vi "Joystick_Operation.vi"(0 "System no.":i32=1 min=1 max=4 step=1, 1 "Joystick ID":u32, 2 "X axis":string="B", 3 "Y axis":string="E", 4 "No.of digits for MOV command":i16=2, 5 "error in":errorcluster, 6 "Resolution factor X":i32=150, 7 "Resolution factor Y":i32=150, 8 "Dead band X":i32=2, 9 "Dead band Y":i32=2, 10 "Use #24 for Stop?":bool=TRUE, 11 "Read from controller?":bool=TRUE caption="Read travel range\nfrom controller?", 12 "Maximum velocity values":T2={"Velocity1 X"=1.0, "Velocity2 X"=20.0, "Velocity1 Y"=0.5, "Velocity2 Y"=15.0} {"Velocity2 Y" format="%.6f"; "Velocity1 Y" format="%.6f"; "Velocity2 X" format="%.6f"; "Velocity1 X" format="%.6f"}, 13 "Travel range":T1={"Xmax"=10.0, "Xmin"=0.0, "Ymax"=5.0, "Ymin"=0.0} {"Ymin" format="%.6f"; "Ymax" format="%.6f"; "Xmin" format="%.6f"; "Xmax" format="%.6f"}, 14 "System no. 2":i32=1 min=1 max=4 step=1) -> (19 "error out":errorcluster)   [LabVIEW 2015]
doc: "This VI can be used to control 2 closed-loop axes (which can belong to one or two connected systems) with a standard 2-button, 2-axis joystick connected to the game port of the host computer. The absolute value of the joystick position is converted into a velocity values for the two stages connected to the system being commanded. Two velocity levels for each axis can be specified, e.g. one for fast, rough positioning and one for slow, fine positioning. Joystick button 2 switches between these levels. The sign of the joystick position determines whether the move command issued contains the positive or negative travel limit (read automatically if Read travel range from controller? is TRUE) of the corresponding axis. When the joystick is \"in the middle position\", the velocity of the corresponding axis is set to zero. \nDead band * is the maximum size of the scaled joystick position value that does not result in any motion. \nResolution factor * determines the joystick resolution. \nNo. of digits is the number of digits after the decimal point in the position values that will be sent by the MOV command. \nIf joystick button 1 is pressed, a stop command (STP or #24, depending on Use 24 for stop, is sent to the controller. The diagram shows how to combine the driver and support VIs for these tasks. \n\nIf only one motion axis is to be controlled, Y Axis must be identical to X Axis, System no. 2 must be identical to System no. 1, and Y axis of joystick is to be used for control of the motion axis.\n\nImportant: Install joystick driver and calibrate joystick in the Windows control panel before running this VI.\n\nValid for C-702, C-843, C-843.PM, C-844, C-848, C-865, C-866, C-867, C-880, E-710, E-712, E-725, E-753, E-755, E-761, E-861\n\nC-702: Use #24 for stop = TRUE, Read from controller = TRUE\n Run \"C702_Configuration_Setup.vi\" prior to running this VI.\n\nC-843: Use #24 for stop = TRUE, Read from controller = TRUE; \n Run \"C843_Configuration_Setup.vi\" prior to running this VI.\n\nC-843.PM: Use #24 for stop = TRUE, Read from controller = TRUE; \n Run \"C843_PM_Configuration_Setup.vi\" prior to running this VI.\n\nC-844: Use #24 for stop = TRUE, Read from controller = TRUE\n Run \"C844_Configuration_Setup.vi\" prior to running this VI.\n\nC-848: Use #24 for stop = TRUE, Read from controller = TRUE\n Run \"C848_Configuration_Setup.vi\" prior to running this VI.\n\nC-865: Use #24 for stop = TRUE, Read from controller = TRUE; \n Run \"C865_Configuration_Setup.vi\" prior to running this VI. \n\nC-866: Use #24 for stop = TRUE, Read from controller = TRUE; \n Run \"C866_Configuration_Setup.vi\" prior to running this VI. \n\nC-867: Use #24 for stop = TRUE, Read from controller = TRUE; \n Run \"C867_Configuration_Setup.vi\" prior to running this VI. \n\nC-880: Use #24 for stop = TRUE, Read from controller = TRUE\n Run \"C880_Configuration_Setup.vi\" prior to running this VI.\n\nE-710: Use #24 for stop = FALSE, Read from controller = TRUE. Default position unit is µm, default velocity unit is µm/ms. Joystick button 1 is not supported (controller does not support #24 or STP). Run \"E710_Configuration_Setup.vi\" prior to running this VI.\n\nE-712: Use #24 for stop = TRUE, Read from controller = TRUE. Default position unit is µm, default velocity unit is µm/s. Run \"E712_Configuration_Setup.vi\" prior to running this VI. \n\nE-725: Use #24 for stop = TRUE, Read from controller = TRUE. Default position unit is µm, default velocity unit is µm/s. Run \"E725_Configuration_Setup.vi\" prior to running this VI. \n\nE-753: Use #24 for stop = TRUE, Read from controller = TRUE. Default position unit is µm, default velocity unit is µm/s. Run \"E753_Configuration_Setup.vi\" prior to running this VI. \n\nE-755: Use #24 for stop = TRUE, Read from controller = TRUE. Default position unit is µm, default velocity unit is µm/s. Run \"E755_Configuration_Setup.vi\" prior to running this VI. VI does not work with E-755.101.\n\nE-761: Use #24 for stop = TRUE, Read from controller = TRUE. Default position unit is µm, default velocity unit is µm/ms. Run \"E761_Configuration_Setup.vi\" prior to running this VI.\n\nE-861: Use #24 for stop = TRUE, Read from controller = TRUE; \n Run \"E861_Configuration_Setup.vi\" prior to running this VI."
panel:
  out "Current Vy":dbl(slide) scale=0.0..0.5 scale format="%.4f"
  out "Current Vx":dbl(slide) scale=0.0..1.0 scale format="%.4f"
  out "Position plot":cluster{dbl[], dbl[]}(graph)
  out "Current pos. Y":dbl format="%.2f"
  out "Current pos. X":dbl format="%.2f"
  out "Current Vy":dbl format="%.6f"
  out "Current Vx":dbl format="%.6f"
  out "Current Vy, max":dbl format="%.6f"
  out "Current Vx, max":dbl format="%.6f"
  in  "stop":bool
  out "JoyY":i32
  out "JoyX":i32
  out "JoyY scaled":i32
  out "JoyX scaled":i32
  # "Joystick operation sample program."
  # "Install joystick driver, calibrate joystick in the Windows control \tpanel and run \"Configuration_Setup.vi\" before running this VI. Use joystick button 1 to stop motion of both\naxes and button2 to switch between two velocity levels. If only one motion axis is to be controlled, Y Axis must be identical to X Axis, System no. 2 must be identical to\nSystem no. 1, and Y axis of joystick is to be used for control of the motion axis.See VI and control/indicator information for details."
  # "For X axis:"
  # "For Y axis:"
  # "Joystick axes settings"
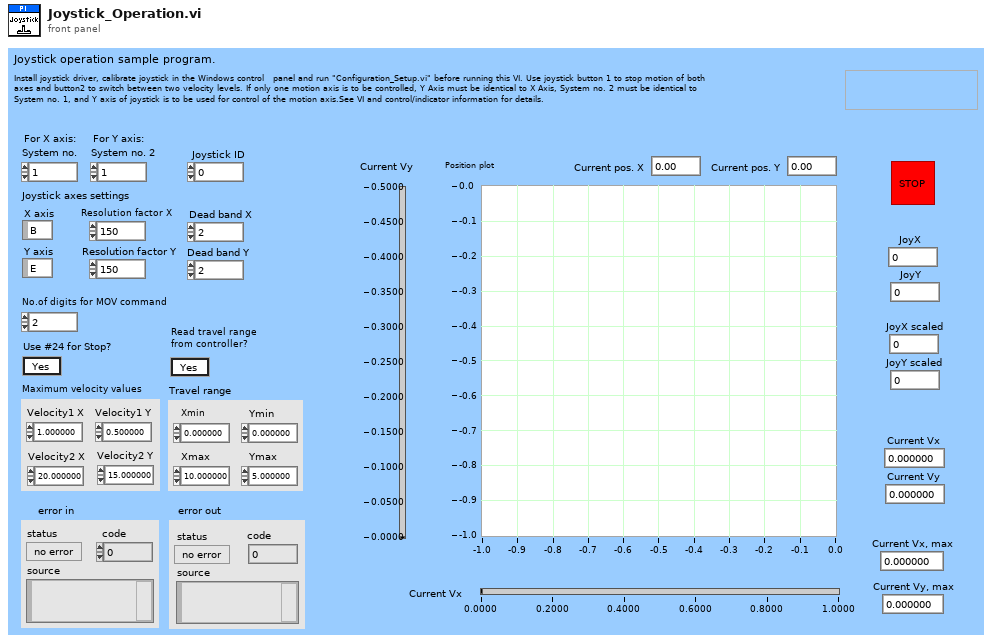
[diagram p1: front panel]
types:
  T1 = cluster{"Xmax":dbl, "Xmin":dbl, "Ymax":dbl, "Ymin":dbl}
  T2 = cluster{"Velocity1 X":dbl, "Velocity2 X":dbl, "Velocity1 Y":dbl, "Velocity2 Y":dbl}
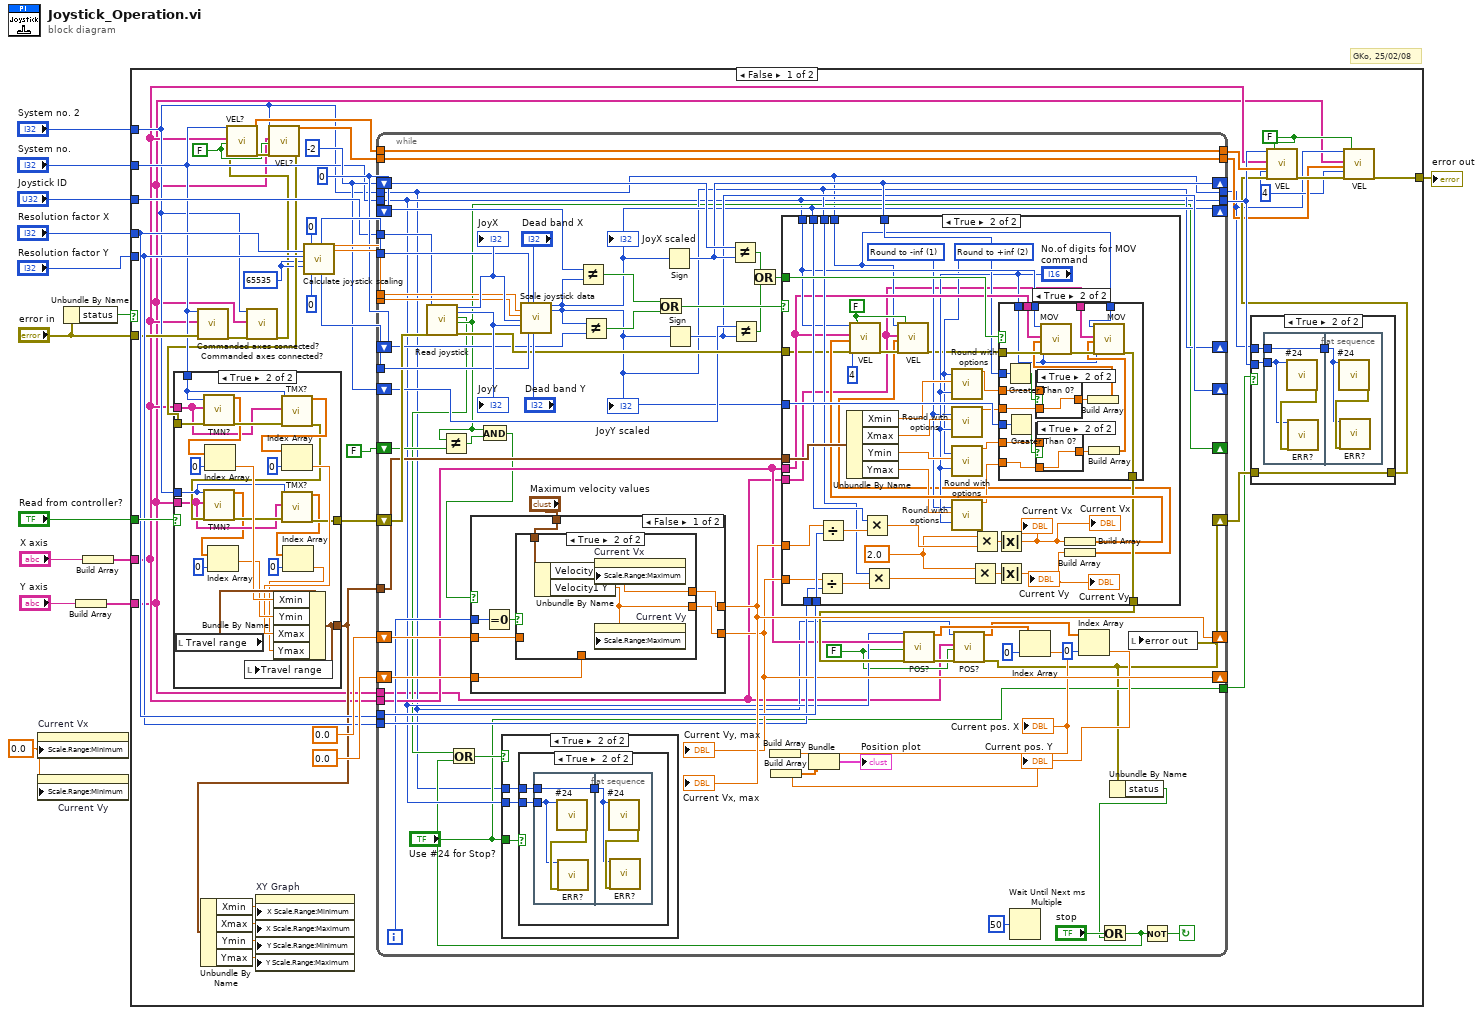
[diagram p0: block diagram]
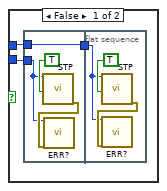
[diagram p7: hidden frame]
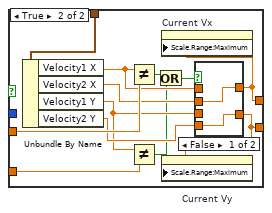
[diagram p9: hidden frame]
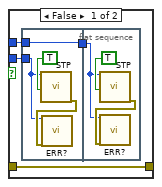
[diagram p11: hidden frame]
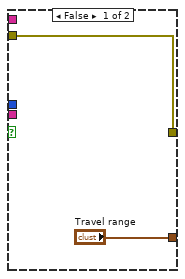
[diagram p12: hidden frame]
diagram:
  w7 = 0.0 ("Write Attribute")
  # "GKo, 25/02/08"
  n1 = property on="Current Vx" class="Slide (strict)"("Scale.Range:Minimum"=w7) -> ()  [unwired: 2 in, 2 out]
  n2 = property on="Current Vy" class="Slide (strict)"("Scale.Range:Minimum"=w7) -> ()  [unwired: 2 in, 2 out]
  n3 = Unbundle By Name("error in") -> ("status"=w9:bool)
  n4 = Build Array("Y axis") -> (w1:string[])
  n5 = Build Array("X axis") -> (w2:string[])
  n6 = case shown="False" w9 {
    tunnel: "Resolution factor X" -> [w46 _]
    tunnel: "Resolution factor Y" -> [w45 _]
    tunnel: "System no." -> [w37 _]
    tunnel: [w19 w287] -> w12
    tunnel: "Read from controller?" -> [w50 _]
    tunnel: "error in" -> [w44 w287]
    tunnel: "Joystick ID" -> [w48 _]
    tunnel: w2 -> [w21 _]
    tunnel: w1 -> [w15 _]
    tunnel: "System no. 2" -> [w22 _]
    frame False {
      w17 = i16 4 ("No.of digits")
      w47 = -2
      w49 = 0 ("XPos scaled")
      w25 = FALSE ("All axes?")
      w30 = FALSE ("Without axis ID?")
      w26 = 65535 ("XPos max")
      n7 = call "Commanded axes connected?.vi"("System no."=w37, "Commanded axes"=w21, "error in"=w44) -> ("error out"=w24:errorcluster)  [unwired: 15 in, 1 out]
      n8 = call "Commanded axes connected?.vi"("System no."=w22, "Commanded axes"=w15, "error in"=w24) -> ("error out"=w23:errorcluster)  [unwired: 15 in, 1 out]
      n9 = call "VEL?.vi"("System no."=w37, "Axes to query"=w21, "All axes?"=w25, "error in"=w23) -> ("Velocity"=w36:dbl[], "error out"=w28:errorcluster)  [unwired: 14 in]
      n10 = call "VEL?.vi"("System no."=w22, "Axes to query"=w15, "All axes?"=w25, "error in"=w28) -> ("Velocity"=w29:dbl[], "error out"=w27:errorcluster)  [unwired: 14 in]
      n11 = case shown="True" w50 {
        tunnel: ["Travel range" w273] -> w43
        tunnel: w27 -> [w262 w285]
        tunnel: [w262 w267] -> w51
        tunnel: w37 -> [_ w284]
        tunnel: w21 -> [_ w272]
        tunnel: w22 -> [_ w270]
        tunnel: w15 -> [_ w266]
        frame False {
        }
        frame True {
          n12 = local read "Travel range"() -> (w279:T1)
          n13 = call "TMN?.vi"("System no."=w284, "Axes to query"=w272, "error in"=w285) -> ("Minimum travel limit"=w283:dbl[], "error out"=w286:errorcluster)  [unwired: 15 in]
          n14 = Index Array(array=w283, index=0 ("Index")) -> (element=w278:dbl)
          n15 = call "TMX?.vi"("System no."=w284, "Axes to query"=w272, "error in"=w286) -> ("Maximum travel limit"=w277:dbl[], "error out"=w269:errorcluster)  [unwired: 15 in]
          n16 = call "TMN?.vi"("System no."=w270, "Axes to query"=w266, "error in"=w269) -> ("Minimum travel limit"=w265:dbl[], "error out"=w268:errorcluster)  [unwired: 15 in]
          n17 = Index Array(array=w265, index=0 ("Index")) -> (element=w276:dbl)
          n18 = Index Array(array=w277, index=0 ("Index")) -> (element=w275:dbl)
          n19 = call "TMX?.vi"("System no."=w270, "Axes to query"=w266, "error in"=w268) -> ("Maximum travel limit"=w264:dbl[], "error out"=w267:errorcluster)  [unwired: 15 in]
          n20 = Index Array(array=w264, index=0 ("Index")) -> (element=w274:dbl)
          n21 = Bundle By Name(cluster=w279, "Xmin"=w278, "Ymin"=w276, "Xmax"=w275, "Ymax"=w274) -> (w273:T1)
          n22 = local write "Travel range"(w273) -> ()
        }
      }
      n23 = Unbundle By Name(w43) -> ("Xmin"=w42:dbl, "Xmax"=w41:dbl, "Ymin"=w40:dbl, "Ymax"=w39:dbl)
      n24 = property on="XY Graph" class="XYGraph (strict)"("X Scale.Range:Minimum"=w42, "X Scale.Range:Maximum"=w41, "Y Scale.Range:Minimum"=w40, "Y Scale.Range:Maximum"=w39) -> ()  [unwired: 2 in, 2 out]
      n25 = call "Calculate joystick scaling.vi"("Resolution factor X"=w46, "Resolution factor Y"=w45, "XPos max"=w26, "YPos max"=w26, "XPos min"=0, "YPos min"=0) -> ("XPos Center scaled"=w57:i32, "YPos Center scaled"=w56:i32, "Scaling factor X"=w55:dbl, "Scaling factor Y"=w54:dbl)  [unwired: 4 in, 6 out]
      n26 = while {
        tunnel: ["Use #24 for Stop?"] -> w31
        tunnel: [w71] -> w35
        tunnel: [w72] -> w33
        tunnel: w36 -> [w71]
        shift-left: FALSE ("Button 2 pressed") -> [w76]
        shift-right: [w74] -> _
        tunnel: w45 -> [w90]
        tunnel: w46 -> [w92]
        shift-left: w47 -> [w98]
        shift-right: [w94] -> _
        shift-left: w47 -> [w99]
        shift-right: [w96] -> _
        tunnel: w48 -> [w103]
        shift-left: w49 -> [w107]
        shift-right: [w89] -> _
        shift-left: w49 -> [w106]
        shift-right: [w88] -> _
        tunnel: w21 -> [w80]
        tunnel: w43 -> [w95]
        shift-left: 0.0 -> [w112]
        shift-right: [w91] -> _
        shift-left: 0.0 -> [w113]
        shift-right: [w93] -> _
        shift-left: w51 -> [w108]
        shift-right: [w64] -> w34
        tunnel: w37 -> [w72]
        tunnel: w54 -> [w117]
        tunnel: w55 -> [w120]
        tunnel: w56 -> [w121]
        tunnel: w57 -> [w122]
        tunnel: w29 -> [w66]
        tunnel: w22 -> [w61]
        tunnel: [w61] -> w16
        tunnel: [w66] -> w18
        tunnel: w15 -> [w60]
        i -> [w87]
        stop <- w116 continue-if-true
        w63 = FALSE ("All axes?")
        n27 = call "Read joystick.vi"("Joystick ID"=w103, "error in"=w108) -> ("XPos"=w124:i32, "YPos"=w123:i32, "Button 1 pressed"=w70:bool, "Button 2 pressed"=w74:bool, "error out"=w109:errorcluster)  [unwired: 13 in]
        "JoyX" <- w124
        "JoyY" <- w123
        n28 = Not Equal?(x=w74, y=w76) -> (x != y?=w75:bool)
        n29 = And(x=w74, y=w75) -> (x .and. y?=w73:bool)
        n30 = case shown="False" w73 {
          tunnel: "Maximum velocity values" -> [w218 w237]
          tunnel: w113 -> [w216 w236]
          tunnel: [w217 w227] -> w93
          tunnel: w112 -> [w214 w231]
          tunnel: [w215 w226] -> w91
          tunnel: w87 -> [w220 _]
          frame False {
            n31 = Equal To 0?(x=w220) -> (x = 0?=w219:bool)
            n32 = case shown="True" w219 {
              tunnel: w218 -> [_ w225]
              tunnel: [w222 w223] -> w217
              tunnel: w216 -> [w222 _]
              tunnel: [w221 w224] -> w215
              tunnel: w214 -> [w221 _]
              frame False {
              }
              frame True {
                n33 = Unbundle By Name(w225) -> ("Velocity1 X"=w223:dbl, "Velocity1 Y"=w224:dbl)
                n34 = property on="Current Vx" class="Slide (strict)"("Scale.Range:Maximum"=w223) -> ()  [unwired: 2 in, 2 out]
                n35 = property on="Current Vy" class="Slide (strict)"("Scale.Range:Maximum"=w224) -> ()  [unwired: 2 in, 2 out]
              }
            }
          }
          frame True {
            n36 = Unbundle By Name(w237) -> ("Velocity1 X"=w235:dbl, "Velocity2 X"=w234:dbl, "Velocity1 Y"=w232:dbl, "Velocity2 Y"=w233:dbl)
            n37 = Not Equal?(x=w235, y=w236) -> (x != y?=w230:bool)
            n38 = Not Equal?(x=w232, y=w231) -> (x != y?=w229:bool)
            n39 = Or(x=w230, y=w229) -> (x .or. y?=w228:bool)
            n40 = case shown="False" w228 {
              tunnel: [w239 w241] -> w227
              tunnel: w235 -> [_ w241]
              tunnel: w234 -> [w239 _]
              tunnel: w233 -> [w238 _]
              tunnel: [w238 w240] -> w226
              tunnel: w232 -> [_ w240]
              frame False {
              }
              frame True {
              }
            }
            n41 = property on="Current Vx" class="Slide (strict)"("Scale.Range:Maximum"=w227) -> ()  [unwired: 2 in, 2 out]
            n42 = property on="Current Vy" class="Slide (strict)"("Scale.Range:Maximum"=w226) -> ()  [unwired: 2 in, 2 out]
          }
        }
        "Current Vx, max" <- w93
        "Current Vy, max" <- w91
        n43 = call "Scale joystick data.vi"("Factor X"=w120, "Factor Y"=w117, "XPos"=w124, "YPos"=w123, "XPos Center"=w122, "YPos Center"=w121, "Dead band X"="Dead band X", "Dead band Y"="Dead band Y") -> ("XPos scaled"=w89:i32, "YPos scaled"=w88:i32)  [unwired: 10 in]
        "JoyX scaled" <- w89
        "JoyY scaled" <- w88
        n44 = Not Equal?(x=w107, y=w89) -> (x != y?=w105:bool)
        n45 = Not Equal?(x=w88, y=w106) -> (x != y?=w104:bool)
        n46 = Or(x=w105, y=w104) -> (x .or. y?=w102:bool)
        n47 = Sign(1:w89) -> (0:w96:i32)
        n48 = Sign(1:w88) -> (0:w94:i32)
        n49 = Not Equal?(x=w99, y=w96) -> (x != y?=w101:bool)
        n50 = Not Equal?(x=w98, y=w94) -> (x != y?=w100:bool)
        n51 = Or(x=w101, y=w100) -> (x .or. y?=w97:bool)
        n52 = case shown="True" w102 {
          tunnel: [w125 w147] -> w84
          tunnel: w109 -> [w125 w145]
          tunnel: w72 -> [_ w149]
          tunnel: w80 -> [_ w148]
          tunnel: w97 -> [_ w166]
          tunnel: w96 -> [_ w144]
          tunnel: w88 -> [_ w165]
          tunnel: w95 -> [_ w164]
          tunnel: w93 -> [_ w163]
          tunnel: w92 -> [_ w162]
          tunnel: w91 -> [_ w161]
          tunnel: w90 -> [_ w160]
          tunnel: w89 -> [_ w157]
          tunnel: w88 -> [_ w156]
          tunnel: w61 -> [_ w127]
          tunnel: w60 -> [_ w126]
          frame False {
          }
          frame True {
            w133 = u16 2 items=["Round to nearest", "Round to -inf", "Round to +inf"] ("Round mode selection")
            w134 = u16 1 items=["Round to nearest", "Round to -inf", "Round to +inf"] ("Round mode selection")
            w150 = 2.0 ("x")
            w130 = FALSE ("Without axis ID?")
            n53 = Divide(x=w161, y=w160) -> (x/y=w158:dbl)
            n54 = Divide(x=w163, y=w162) -> (x/y=w159:dbl)
            n55 = Unbundle By Name(w164) -> ("Xmin"=w143:dbl, "Xmax"=w141:dbl, "Ymin"=w139:dbl, "Ymax"=w137:dbl)
            n56 = Multiply(x=w157, y=w159) -> (x*y=w155:dbl)
            n57 = Multiply(x=w156, y=w158) -> (x*y=w154:dbl)
            n58 = call "Round with options.vi"("Round mode selection"=w133, "Numeric in"=w143, "No.of digits\nto round to"="No.of digits for MOV command") -> ("Numeric out"=w142:dbl)  [unwired: 15 in, 1 out]
            n59 = call "Round with options.vi"("Round mode selection"=w134, "Numeric in"=w141, "No.of digits\nto round to"="No.of digits for MOV command") -> ("Numeric out"=w140:dbl)  [unwired: 15 in, 1 out]
            n60 = call "Round with options.vi"("Round mode selection"=w133, "Numeric in"=w139, "No.of digits\nto round to"="No.of digits for MOV command") -> ("Numeric out"=w138:dbl)  [unwired: 15 in, 1 out]
            n61 = call "Round with options.vi"("Round mode selection"=w134, "Numeric in"=w137, "No.of digits\nto round to"="No.of digits for MOV command") -> ("Numeric out"=w136:dbl)  [unwired: 15 in, 1 out]
            n62 = Multiply(x=w150, y=w154) -> (x*y=w151:dbl)
            n63 = Multiply(x=w150, y=w155) -> (x*y=w152:dbl)
            n64 = Absolute Value(x=w152) -> (abs(x)=w146:dbl)
            "Current Vx" <- w146
            "Current Vx" <- w146
            n65 = Absolute Value(x=w151) -> (abs(x)=w129:dbl)
            "Current Vy" <- w129
            "Current Vy" <- w129
            n66 = Build Array(w146) -> (w153:dbl[])
            n67 = call "VEL.vi"("System no."=w149, "Axes to set"=w148, "Velocity values"=w153, "No.of digits"=i16 4, "error in"=w145, "Without axis ID?"=w130) -> ("error out"=w132:errorcluster)  [unwired: 12 in, 1 out]
            n68 = Build Array(w129) -> (w128:dbl[])
            n69 = call "VEL.vi"("System no."=w127, "Axes to set"=w126, "Velocity values"=w128, "error in"=w132, "Without axis ID?"=w130) -> ("error out"=w131:errorcluster)  [unwired: 13 in, 1 out]
            n70 = case shown="True" w166 {
              tunnel: [w168 w173] -> w147
              tunnel: "No.of digits for MOV command" -> [_ w169]
              tunnel: w131 -> [w168 w188]
              tunnel: w149 -> [_ w187]
              tunnel: w148 -> [_ w186]
              tunnel: w144 -> [_ w185]
              tunnel: w165 -> [_ w184]
              tunnel: w140 -> [_ w182]
              tunnel: w142 -> [_ w181]
              tunnel: w138 -> [_ w179]
              tunnel: w136 -> [_ w178]
              tunnel: w127 -> [_ w172]
              tunnel: w126 -> [_ w171]
              frame False {
              }
              frame True {
                n71 = Greater Than 0?(x=w185) -> (x > 0?=w183:bool)
                n72 = Greater Than 0?(x=w184) -> (x > 0?=w180:bool)
                n73 = case shown="True" w183 {
                  tunnel: w182 -> [_ w192]
                  tunnel: w181 -> [w191 _]
                  tunnel: [w191 w192] -> w177
                  frame False {
                  }
                  frame True {
                  }
                }
                n74 = case shown="True" w180 {
                  tunnel: w179 -> [w189 _]
                  tunnel: w178 -> [_ w190]
                  tunnel: [w189 w190] -> w175
                  frame False {
                  }
                  frame True {
                  }
                }
                n75 = Build Array(w177) -> (w176:dbl[])
                n76 = call "MOV.vi"("System no."=w187, "Axes to move"=w186, "Position values"=w176, "No.of digits"=w169, "error in"=w188) -> ("error out"=w174:errorcluster)  [unwired: 14 in]
                n77 = Build Array(w175) -> (w170:dbl[])
                n78 = call "MOV.vi"("System no."=w172, "Axes to move"=w171, "Position values"=w170, "No.of digits"=w169, "error in"=w174) -> ("error out"=w173:errorcluster)  [unwired: 14 in]
              }
            }
          }
        }
        n79 = call "POS?.vi"("System no."=w72, "Axes to query"=w80, "All axes?"=w63, "error in"=w84) -> ("Position"=w83:dbl[], "error out"=w65:errorcluster)  [unwired: 14 in]
        n80 = call "POS?.vi"("System no."=w61, "Axes to query"=w60, "All axes?"=w63, "error in"=w65) -> ("Position"=w62:dbl[], "error out"=w64:errorcluster)  [unwired: 14 in]
        n81 = Wait Until Next ms Multiple(millisecond multiple=u32 50) -> ()  [unwired: 1 out]
        n82 = Index Array(array=w83, index=0 ("Index")) -> (element=w82:dbl)
        "Current pos. X" <- w82
        n83 = Build Array(w82) -> (w79:dbl[])
        n84 = Index Array(array=w62, index=0 ("Index")) -> (element=w81:dbl)
        "Current pos. Y" <- w81
        n85 = Build Array(w81) -> (w78:dbl[])
        n86 = Bundle(w79, w78) -> (→"Position plot":cluster{dbl[], dbl[]})  [unwired: 1 in]
        n87 = Unbundle By Name(w64) -> ("status"=w110:bool)
        n88 = Or(x="stop", y=w110) -> (x .or. y?=w69:bool)
        n89 = Or(x=w70, y=w69) -> (x .or. y?=w68:bool)
        n90 = case shown="True" w68 {
          tunnel: w72 -> [_ w195]
          tunnel: "Use #24 for Stop?" -> [_ w194]
          tunnel: w61 -> [_ w193]
          frame False {
          }
          frame True {
            n91 = case shown="True" w194 {
              tunnel: w195 -> [w197 w206]
              tunnel: w193 -> [w196 w207]
              frame False {
                n92 = flat-sequence {
                  tunnel: w196 -> [w199]
                  tunnel: [w199] -> w198
                  tunnel: w197 -> [w200]
                  tunnel: w198 -> [w203]
                  frame #0 {
                    n93 = call "STP.vi"("System no."=w200, "All axes?"=TRUE) -> ("error out"=w202:errorcluster)  [unwired: 17 in]
                    n94 = call "ERR?.vi"("System no."=w200, "error in"=w202) -> ()  [unwired: 16 in, 2 out]
                  }
                  frame #1 {
                    n95 = call "STP.vi"("System no."=w203, "All axes?"=TRUE) -> ("error out"=w204:errorcluster)  [unwired: 17 in]
                    n96 = call "ERR?.vi"("System no."=w203, "error in"=w204) -> ()  [unwired: 16 in, 2 out]
                  }
                }
              }
              frame True {
                n97 = flat-sequence {
                  tunnel: w207 -> [w210]
                  tunnel: [w210] -> w208
                  tunnel: w206 -> [w209]
                  tunnel: w208 -> [w212]
                  frame #0 {
                    n98 = call "#24.vi"("System no."=w209) -> ("error out"=w211:errorcluster)  [unwired: 18 in]
                    n99 = call "ERR?.vi"("System no."=w209, "error in"=w211) -> ()  [unwired: 16 in, 2 out]
                  }
                  frame #1 {
                    n100 = call "#24.vi"("System no."=w212) -> ("error out"=w213:errorcluster)  [unwired: 18 in]
                    n101 = call "ERR?.vi"("System no."=w212, "error in"=w213) -> ()  [unwired: 16 in, 2 out]
                  }
                }
              }
            }
          }
        }
        n102 = local write "error out"(w64) -> ()
        n103 = Not(x=w69) -> (.not. x?=w116:bool)
      }
      n104 = case shown="True" w31 {
        tunnel: w33 -> [w242 w253]
        tunnel: w34 -> [w245 w256]
        tunnel: [w245 w256] -> w32
        tunnel: w16 -> [w244 w255]
        frame False {
          n105 = flat-sequence {
            tunnel: w244 -> [w247]
            tunnel: [w247] -> w243
            tunnel: w242 -> [w246]
            tunnel: w243 -> [w250]
            frame #0 {
              n106 = call "STP.vi"("System no."=w246, "All axes?"=TRUE) -> ("error out"=w249:errorcluster)  [unwired: 17 in]
              n107 = call "ERR?.vi"("System no."=w246, "error in"=w249) -> ()  [unwired: 16 in, 2 out]
            }
            frame #1 {
              n108 = call "STP.vi"("System no."=w250, "All axes?"=TRUE) -> ("error out"=w251:errorcluster)  [unwired: 17 in]
              n109 = call "ERR?.vi"("System no."=w250, "error in"=w251) -> ()  [unwired: 16 in, 2 out]
            }
          }
        }
        frame True {
          n110 = flat-sequence {
            tunnel: w255 -> [w258]
            tunnel: [w258] -> w254
            tunnel: w253 -> [w257]
            tunnel: w254 -> [w260]
            frame #0 {
              n111 = call "#24.vi"("System no."=w257) -> ("error out"=w259:errorcluster)  [unwired: 18 in]
              n112 = call "ERR?.vi"("System no."=w257, "error in"=w259) -> ()  [unwired: 16 in, 2 out]
            }
            frame #1 {
              n113 = call "#24.vi"("System no."=w260) -> ("error out"=w261:errorcluster)  [unwired: 18 in]
              n114 = call "ERR?.vi"("System no."=w260, "error in"=w261) -> ()  [unwired: 16 in, 2 out]
            }
          }
        }
      }
      n115 = call "VEL.vi"("System no."=w33, "Axes to set"=w21, "Velocity values"=w35, "No.of digits"=w17, "error in"=w32, "Without axis ID?"=w30) -> ("error out"=w20:errorcluster)  [unwired: 12 in, 1 out]
      n116 = call "VEL.vi"("System no."=w16, "Axes to set"=w15, "Velocity values"=w18, "No.of digits"=w17, "error in"=w20, "Without axis ID?"=w30) -> ("error out"=w19:errorcluster)  [unwired: 12 in, 1 out]
    }
    frame True {
    }
  }
  "error out" <- w12
